vi "Write Version.vi"(8 "error in (no error)":errorcluster, 10 "Version":string, 11 "Lib in":refnum<class "Lib.lvclass">) -> (0 "error out":errorcluster, 3 "Lib out":refnum<class "Lib.lvclass">)   [LabVIEW 2021, in "TAF Proj Document Type.lvlib" / "Lib.lvclass"]
uses:
  <vilib>/Wovalab/AntiDoc/Document Type/Add-ons/LabVIEW TAF Project/Lib/Lib.lvclass
  <vilib>/Wovalab/AntiDoc/Document Type/Add-ons/LabVIEW TAF Project/Lib/Lib.lvclass/Lib.ctl
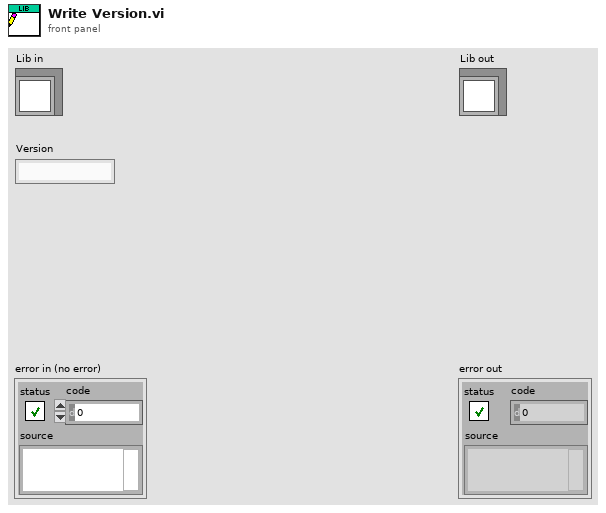
[diagram p1: front panel]
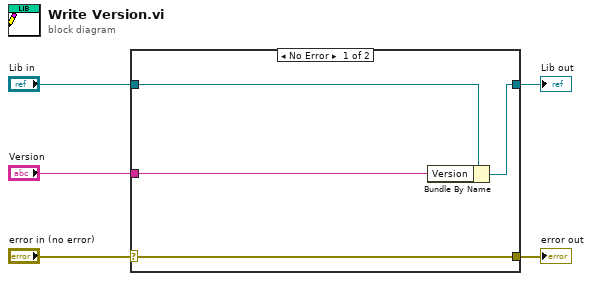
[diagram p0: block diagram]
diagram:
  n1 = case shown="No Error" "error in (no error)" {
    selector: "error in (no error)" -> [w9 w10]
    tunnel: [w9 w10] -> w4
    tunnel: [w7 w11] -> w2
    tunnel: "Lib in" -> [w8 w11]
    tunnel: "Version" -> [w6 _]
    frame No Error {
      n2 = Bundle By Name(cluster=w8, "Version"=w6) -> (w7:refnum<class "Lib.lvclass">)
    }
    frame Error {
    }
  }
  "error out" <- w4
  "Lib out" <- w2
